vi "8Pixel.vi"() -> (3 "8 pixel":u32)   [LabVIEW 2009, in "menu item.lvclass"]
uses:
  menu item.lvclass
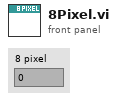
[diagram p1: front panel]
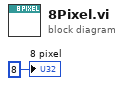
[diagram p0: block diagram]
diagram:
  "8 pixel" <- u32 8 ("1 pixel")
